vi "SetParam.vi"(8 "error in (no error)":errorcluster caption="entrée d'erreur (pas d'erreur)", 10 "cosine_similarity":cluster{"dense_output":bool}={"dense_output"=TRUE}, 11 "Cosine_similarity.lvclass":refnum<class "Cosine_similarity.lvclass">) -> (0 "error out":errorcluster caption="sortie d'erreur", 3 "Cosine_similarity.lvclass":refnum<class "Cosine_similarity.lvclass">)   [LabVIEW 2020, in "Cosine_similarity.lvclass"]
doc: "Set Parameters"
uses:
  Cosine_similarity.lvclass
  Cosine_similarity.lvclass/Cosine_similarity.ctl
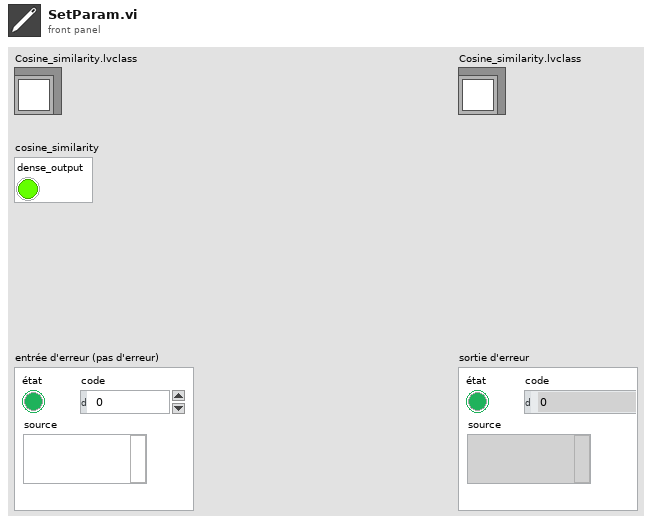
[diagram p1: front panel]
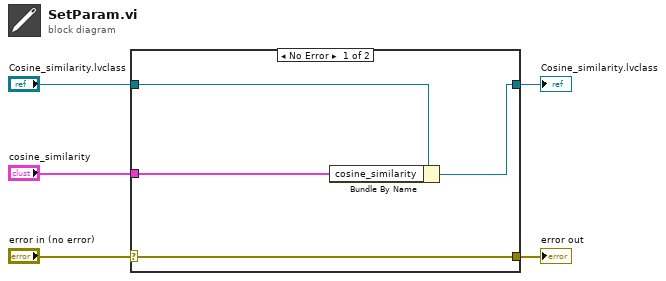
[diagram p0: block diagram]
diagram:
  n1 = case shown="No Error" "error in (no error)" {
    selector: "error in (no error)" -> [w9 w10]
    tunnel: [w9 w10] -> w4
    tunnel: [w7 w11] -> w2
    tunnel: "Cosine_similarity.lvclass" -> [w8 w11]
    tunnel: "cosine_similarity" -> [w6 _]
    frame No Error {
      n2 = Bundle By Name(cluster=w8, "cosine_similarity"=w6) -> (w7:refnum<class "Cosine_similarity.lvclass">)
    }
    frame Error {
    }
  }
  "error out" <- w4
  "Cosine_similarity.lvclass" <- w2
